vi "Global 1.vi"() -> ()   [LabVIEW 2017]
panel:
  in  "data value reference":refnum<data-value>
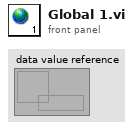
[diagram p1: front panel]
diagram:
